vi "MD5 Hash__ogtk.vi"(1 "Strict Case? (False)":bool, 3 "Input String":string) -> (0 "MD5 Hash?":bool)   [LabVIEW 2020]
doc: "<b>MD5 Hash?</b> returns TRUE if <b>Input String</b> represents an MD5 Hash otherwise, it returns FALSE.\n\nFor a valid Hash the <b>Input String</b> should be 32 characters and consist of the following characters: 0-9, a-f or A-F. \nE.g. \"6a204bd89f3c8348afd5c77c717a097a\" or \"6A204BD89F3C8348AFD5C77C717A097A\"\n\nIf <b>Strict Case</b> = TRUE, <b>Input String</b> should only consist of the following characters: 0-9 or a-f.\nE.g. \"6a204bd89f3c8348afd5c77c717a097a\""
panel:
  # "Please visit http://www.OpenG.org to learn about the\nOpen Source LabVIEW software movement.\n\nNOTICE -- YOU MUST LEAVE THIS NOTICE IN PLACE.  PER THE TERMS OF THE LICENSE BELOW, YOU MAY SUBLICENSE THIS SOFTWARE \nIN ANY WAY THAT DOES NOT CONFLICT WITH THIS LICENSE.\n\n### BSD License (http://www.opensource.org/licenses/bsd-license.php) Begin ###\n \nCopyright (c) 2011, Chris Beuschel <cbeuschel@viengineering.com>\nCopyright (c) 2011, Jonathon Green <jg@jgcode.net>\n\nAll rights reserved.\n\nRedistribution and use in source and binary forms, with or without modification, are permitted provided that the following conditions are met:\n\n    * Redistributions of source code must retain the above copyright notice, this list of conditions and the following disclaimer.\n    * Redistributions in binary form must reproduce the above copyright notice, this list of conditions and the following disclaimer in the \n       documentation and/or other materials provided with the distribution.\n    * Neither the name of SciWare, James Kring, Inc., nor the names of its contributors may be used to endorse or promote products derived \n       from this software without specific prior written permission.\n\nTHIS SOFTWARE IS PROVIDED BY THE COPYRIGHT HOLDERS AND CONTRIBUTORS \"AS IS\" AND ANY EXPRESS OR IMPLIED WARRANTIES, \nINCLUDING, BUT NOT LIMITED TO, THE IMPLIED WARRANTIES OF MERCHANTABILITY AND FITNESS FOR A PARTICULAR PURPOSE ARE \nDISCLAIMED. IN NO EVENT SHALL THE COPYRIGHT OWNER OR CONTRIBUTORS BE LIABLE FOR ANY DIRECT, INDIRECT, INCIDENTAL,\n SPECIAL, EXEMPLARY, OR CONSEQUENTIAL DAMAGES (INCLUDING, BUT NOT LIMITED TO, PROCUREMENT OF SUBSTITUTE GOODS OR \nSERVICES; LOSS OF USE, DATA, OR PROFITS; OR BUSINESS INTERRUPTION) HOWEVER CAUSED AND ON ANY THEORY OF LIABILITY, \nWHETHER IN CONTRACT, STRICT LIABILITY, OR TORT (INCLUDING NEGLIGENCE OR OTHERWISE) ARISING IN ANY WAY OUT OF THE USE \nOF THIS SOFTWARE, EVEN IF ADVISED OF THE POSSIBILITY OF SUCH DAMAGE.\n\n### BSD License End ###"
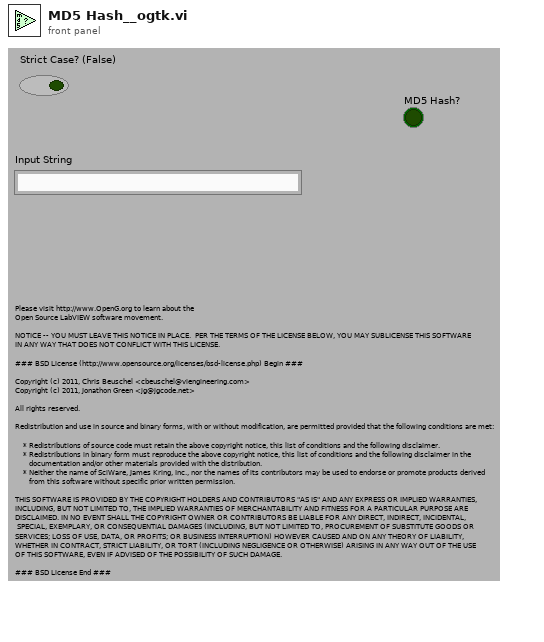
[diagram p1: front panel]
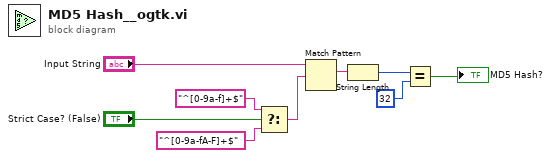
[diagram p0: block diagram]
diagram:
  n1 = Select(t="^[0-9a-f]+$" ("regular expression"), s="Strict Case? (False)", f="^[0-9a-fA-F]+$" ("regular expression")) -> (s? t:f=w3:string)
  n2 = Match Pattern(string="Input String", regular expression=w3) -> (match substring=w7:string)  [unwired: 1 in, 3 out]
  n3 = String Length(string=w7) -> (length=w9:i32)
  n4 = Equal?(x=w9, y=32 ("x")) -> (x = y?=→"MD5 Hash?":bool)
